vi "PrepareNumerator.vi"(0 "A":T1={"Array Num"=[1, 2, 3], "Decimal Index"=0, "stop"=FALSE}, 1 "B":T1={"Array Num"=[1, 2, 3], "Decimal Index"=0, "stop"=FALSE}) -> (2 "Normalized A":T1={"Array Num"=[1, 2, 3], "Decimal Index"=0, "stop"=FALSE}, 3 "B copy":T1={"Array Num"=[1, 2, 3], "Decimal Index"=0, "stop"=FALSE}, 4 "Shifted":i32)   [LabVIEW 2025]
doc: "Make sure Numerator is less than denominators"
uses:
  Number.ctl
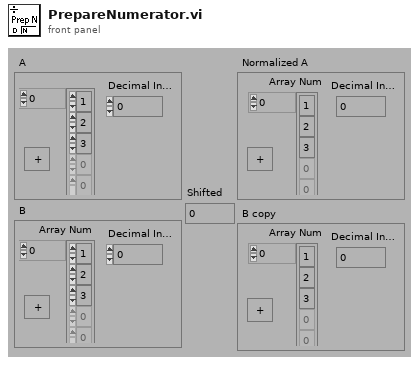
[diagram p1: front panel]
types:
  T1 = typedef "Number.ctl" = cluster{"Array Num":i8[], "Decimal Index":i32, "stop":bool}
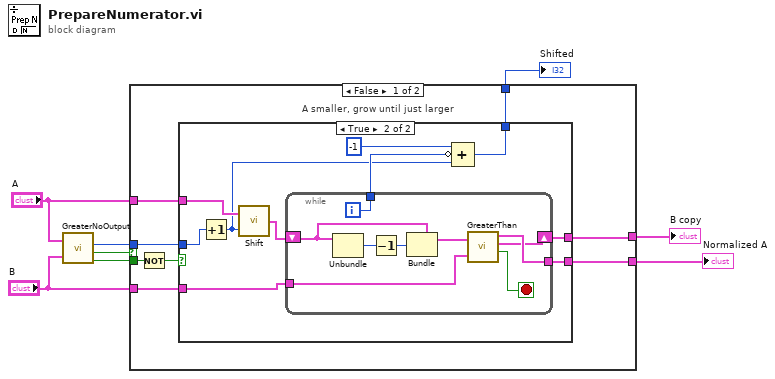
[diagram p0: block diagram]
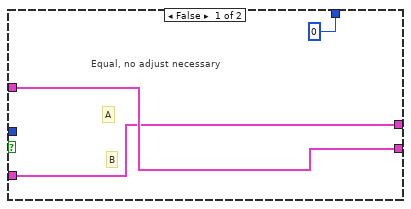
[diagram p2: hidden frame]
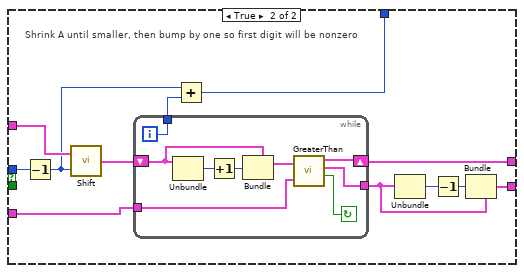
[diagram p3: hidden frame]
diagram:
  n1 = call "GreaterNoOutput.vi"("A"="A", "B"="B") -> ("Digit Shift"=w1:i32, "A Greater"=w8:bool, "Equal"=w4:bool)  [unwired: 1 in]
  n2 = case shown="False" w8 {
    tunnel: [w13 w48] -> w5
    tunnel: [w16 w40] -> w7
    tunnel: [w14 w50] -> w6
    tunnel: w4 -> [w15 _]
    tunnel: "A" -> [w10 w43]
    tunnel: "B" -> [w11 w45]
    tunnel: w1 -> [w9 w44]
    frame False {
      # "A smaller, grow until just larger"
      n3 = Not(x=w15) -> (.not. x?=w12:bool)
      n4 = case shown="True" w12 {
        tunnel: [w17 w29] -> w14
        tunnel: [w18 w28] -> w13
        tunnel: [0 w20] -> w16
        tunnel: w10 -> [w18 w26]
        tunnel: w11 -> [w17 w27]
        tunnel: w9 -> [_ w24]
        frame False {
          # "B"
          # "A"
          # "Equal, no adjust necessary"
        }
        frame True {
          n5 = Increment(x=w24) -> (x+1=w21:i32)
          n6 = call "Shift.vi"("Shift by"=w21, "A"=w26) -> ("Shifted A"=w25:T1)
          n7 = while {
            tunnel: [w37] -> w22
            tunnel: [w35] -> w28
            shift-left: w25 -> [w30]
            shift-right: [w34] -> w29
            tunnel: w27 -> [w36]
            i -> [w37]
            stop <- w38 stop-if-true
            n8 = Unbundle(w30) -> ("Decimal Index"=w32:i32)  [unwired: 2 out]
            n9 = Decrement(x=w32) -> (x-1=w33:i32)
            n10 = Bundle(cluster=w30, "Decimal Index"=w33) -> (w31:T1)  [unwired: 2 in]
            n11 = call "GreaterThan.vi"("A"=w31, "B"=w36) -> ("Larger"=w35:T1, "Smaller"=w34:T1, "A Greater"=w38:bool)  [unwired: 1 out]
          }
          n12 = Compound Arithmetic op=ADD(-1, invert w22, w21) -> (w20:i32)
        }
      }
    }
    frame True {
      # "Shrink A until smaller, then bump by one so first digit will be nonzero"
      n13 = Decrement(x=w44) -> (x-1=w41:i32)
      n14 = call "Shift.vi"("Shift by"=w41, "A"=w43) -> ("Shifted A"=w42:T1)
      n15 = while {
        tunnel: [w56] -> w39
        tunnel: [w57] -> w49
        shift-left: w42 -> [w52]
        shift-right: [w58] -> w50
        tunnel: w45 -> [w55]
        i -> [w56]
        stop <- w59 continue-if-true
        n16 = Unbundle(w52) -> ("Decimal Index"=w53:i32)  [unwired: 2 out]
        n17 = Increment(x=w53) -> (x+1=w54:i32)
        n18 = Bundle(cluster=w52, "Decimal Index"=w54) -> (w51:T1)  [unwired: 2 in]
        n19 = call "GreaterThan.vi"("A"=w51, "B"=w55) -> ("Larger"=w58:T1, "Smaller"=w57:T1, "A Greater"=w59:bool)  [unwired: 1 out]
      }
      n20 = Add(x=w41, y=w39) -> (x+y=w40:i32)
      n21 = Unbundle(w49) -> ("Decimal Index"=w46:i32)  [unwired: 2 out]
      n22 = Decrement(x=w46) -> (x-1=w47:i32)
      n23 = Bundle(cluster=w49, "Decimal Index"=w47) -> (w48:T1)  [unwired: 2 in]
    }
  }
  "Normalized A" <- w5
  "Shifted" <- w7
  "B copy" <- w6
